vi "Gimbal 3.vi"(2 "frequency (periods/tick)":fxp<+,32,0>, 5 "PITCH 3":fxp<+,32,0>, 9 "ROLL 3":fxp<+,32,0>, 11 "YAW 3":fxp<+,32,0>) -> (4 "DIO 13":bool, 6 "DIO 14":bool, 15 "DIO 15":bool)   [LabVIEW 2015]
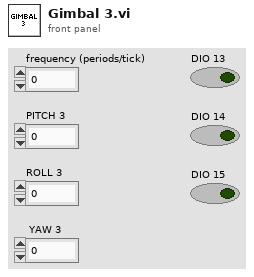
[diagram p1: front panel]
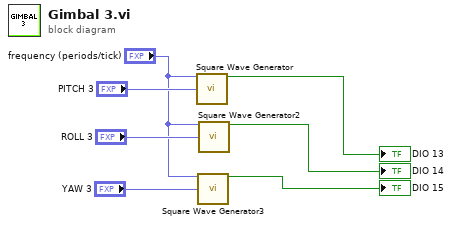
[diagram p0: block diagram]
diagram:
  n1 = call "Square Wave Generator"("frequency (periods/tick)"="frequency (periods/tick)", "duty cycle (periods)"="PITCH 3") -> ("square wave out"=→"DIO 13":bool)  [unwired: 13 in]
  n2 = call "Square Wave Generator3"("frequency (periods/tick)"="frequency (periods/tick)", "duty cycle (periods)"="YAW 3") -> ("square wave out"=→"DIO 15":bool)  [unwired: 13 in]
  n3 = call "Square Wave Generator2"("frequency (periods/tick)"="frequency (periods/tick)", "duty cycle (periods)"="ROLL 3") -> ("square wave out"=→"DIO 14":bool)  [unwired: 13 in]
